vi "GoTo Read.vi"(8 "error in (no error)":errorcluster caption="entrée d'erreur (pas d'erreur)", 11 "Class UART Enocean en entrée":refnum<class "Class UART Enocean.lvclass">) -> (0 "error out":errorcluster caption="sortie d'erreur", 3 "Class UART Enocean en sortie":refnum<class "Class UART Enocean.lvclass">)   [LabVIEW 2020, in "Library Instrument & Equipement.lvlib" / "Library UART.lvlib" / "Class UART Enocean.lvclass"]
uses:
  Class UART Enocean.lvclass
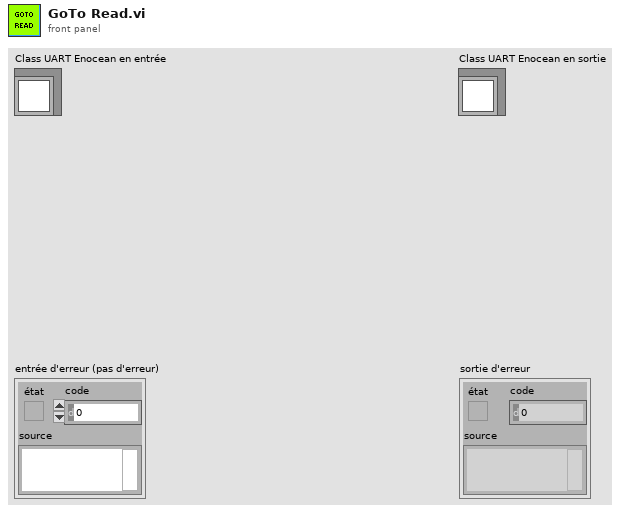
[diagram p1: front panel]
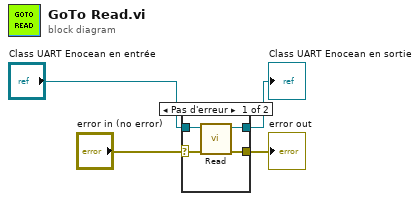
[diagram p0: block diagram]
diagram:
  n1 = case shown="Pas d'erreur" "error in (no error)" {
    selector: "error in (no error)" -> [w6 w10]
    tunnel: [w5 w10] -> w3
    tunnel: [w7 w9] -> w1
    tunnel: "Class UART Enocean en entrée" -> [w8 w9]
    frame No Error {
      n2 = call-dynamic "Read.vi"("error in (no error)"=w6, "Class UART (Default) en entrée"=w8) -> ("error out"=w5:errorcluster, "Class UART (Default) en sortie"=w7:refnum<class "Class UART Enocean.lvclass">)  [unwired: 8 in]
    }
    frame Error {
    }
  }
  "error out" <- w3
  "Class UART Enocean en sortie" <- w1
